vi "Read Sequence parameters.vi"() -> (20 "Software_ID":string, 21 "Software_Version":string, 22 "Bootloader_ID":string, 23 "Bootloader_Version":string, 24 "Calibration_Release_Number_0":string, 25 "Calibration_Release_Number_1":string, 26 "Calibration_Release_Number_2":string, 27 "error out":errorcluster)   [LabVIEW 2025]
uses:
  <vilib>/Utility/config.llb/Read Key (String).vi
  <vilib>/Utility/config.llb/NI_LVConfig.lvlib
panel:
  out "Parameter values":string[](array[string])
  out "Parameters":string[](array[string])
  in  "error in (no error)":errorcluster
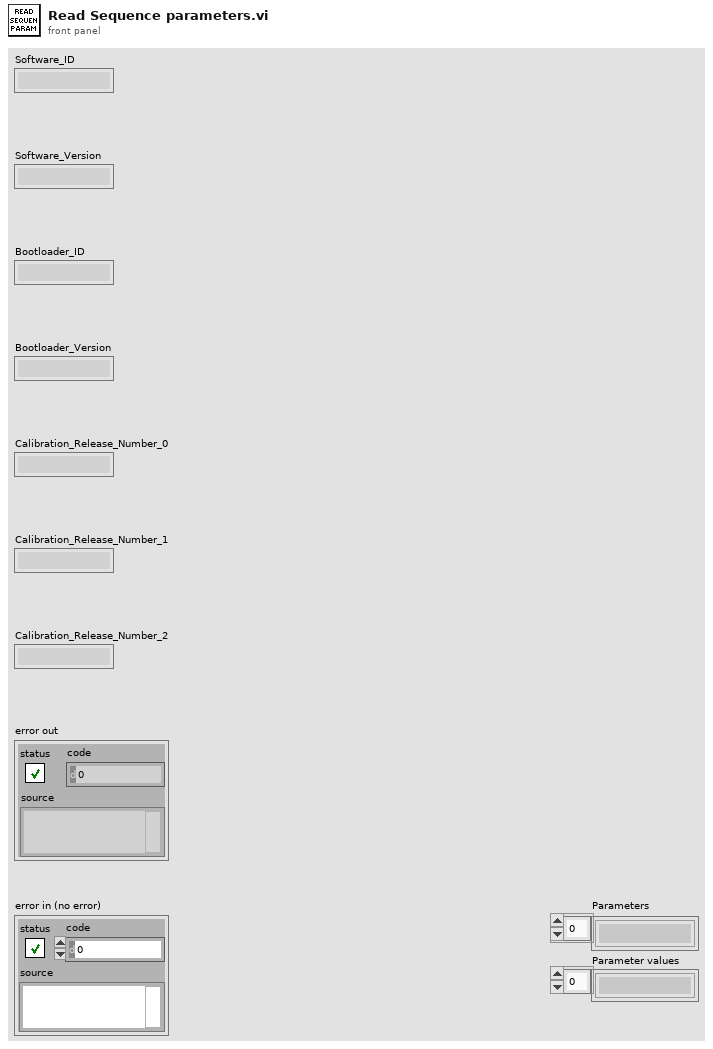
[diagram p1: front panel]
types:
  T1 = typedef "NI_LVConfig.lvlib/Config Data RefNum.ctl" = refnum<k1>
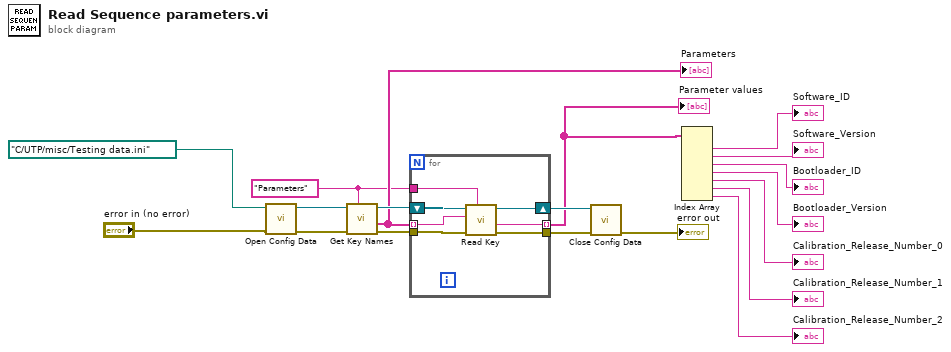
[diagram p0: block diagram]
diagram:
  w1 = "Parameters" ("section")
  n1 = call <vilib>:"Open Config Data.vi"("error in (no error)"="error in (no error)", "configuration file path"=path "C:/UTP/misc/Testing data.ini") -> ("error out"=w15:errorcluster, "refnum"=w17:T1)  [unwired: 7 in, 1 out]
  n2 = call <vilib>:"Get Key Names.vi"("section"=w1, "error in (no error)"=w15, "refnum"=w17) -> ("error out"=w14:errorcluster, "key names"=w13:string[], "refnum out"=w16:T1)  [unwired: 5 in, 1 out]
  "Parameters" <- w13
  n3 = for {
    tunnel: w14 -> [w25]
    tunnel: w13 -> [w24] mode=indexing
    tunnel: [w23] -> w10 mode=indexing
    shift-right: [w22] -> w12
    shift-left: w16 -> [w26]
    tunnel: [w21] -> w11
    tunnel: w1 -> [w20]
    n4 = call-poly <vilib>:"Read Key.vi"("section"=w20, "error in (no error)"=w25, "key"=w24, "refnum"=w26) -> ("error out"=w21:errorcluster, "value"=w23:string, "refnum out"=w22:T1)  [unwired: 4 in, 1 out]
  }
  "Parameter values" <- w10
  n5 = call <vilib>:"Close Config Data.vi"("error in (no error)"=w11, "refnum"=w12) -> ("error out"=→"error out":errorcluster)  [unwired: 8 in, 1 out]
  n6 = Index Array(array=w10) -> (element #1=→"Software_ID":string, element #2=→"Software_Version":string, element #3=→"Bootloader_ID":string, element #4=→"Bootloader_Version":string, element #5=→"Calibration_Release_Number_0":string, element #6=→"Calibration_Release_Number_1":string, element #7=→"Calibration_Release_Number_2":string)  [unwired: 7 in]
